vi "Write Trigger.vi"(8 "error in (no error)":errorcluster, 10 "PV":refnum<class "PV.lvclass">, 11 "PVConnection in":refnum<class "PVConnection.lvclass">) -> (0 "error out":errorcluster, 3 "PVConnection out":refnum<class "PVConnection.lvclass">)   [LabVIEW 2015, in "CS++ProcessVariables.lvlib" / "PVConnection.lvclass"]
doc: "Publish a process variable to trigger a paramater less message."
uses:
  PVConnection.lvclass
  ProcessVariable/PV.lvclass
  PVConnection.lvclass/PVConnection.ctl
  ProcessVariable/PV.lvclass/PV.ctl
  CS++BaseClasses/Base/CS++Base.lvclass/CS++Base.ctl
  Libraries/Utilities/CS++Utilities.lvlib
  CS++BaseClasses/Base/CS++Base.lvclass
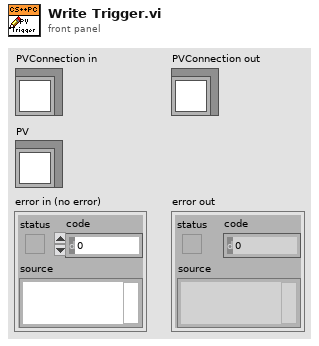
[diagram p1: front panel]
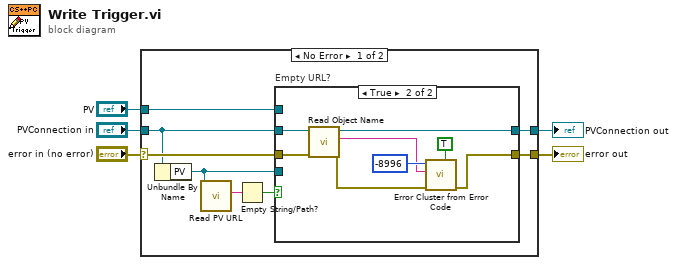
[diagram p0: block diagram]
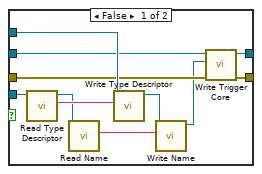
[diagram p2: hidden frame]
diagram:
  n1 = case shown="No Error" "error in (no error)" {
    selector: "error in (no error)" -> [w12 w34]
    tunnel: [w9 w34] -> w4
    tunnel: [w10 w33] -> w2
    tunnel: "PVConnection in" -> [w11 w33]
    tunnel: "PV" -> [w13 _]
    frame No Error {
      n2 = Unbundle By Name(w11) -> ("PV"=w7:refnum<class "PV.lvclass">)
      n3 = call "Read PV URL.vi"("PV in"=w7) -> ("PV URL"=w8:string)  [unwired: 8 in, 2 out]
      n4 = Empty String/Path?(string/path=w8) -> (empty?=w6:bool)
      n5 = case "Empty URL?" shown="True" w6 {
        tunnel: w13 -> [w24 _]
        tunnel: w12 -> [w19 w27]
        tunnel: w11 -> [w17 w29]
        tunnel: [w16 w28] -> w10
        tunnel: [w15 w30] -> w9
        tunnel: w7 -> [w14 _]
        frame False {
          n6 = call "Read Type Descriptor.vi"("PV in"=w14) -> ("Type Descriptor"=w23:string, "PV out"=w22:refnum<class "PV.lvclass">)  [unwired: 8 in, 1 out]
          n7 = call "Read Name.vi"("PV in"=w22) -> ("Name"=w21:string)  [unwired: 8 in, 2 out]
          n8 = call "Write Type Descriptor.vi"("Type Descriptor"=w23, "PV in"=w24) -> ("PV out"=w20:refnum<class "PV.lvclass">)  [unwired: 8 in, 1 out]
          n9 = call "Write Name.vi"("Name"=w21, "PV in"=w20) -> ("PV out"=w18:refnum<class "PV.lvclass">)  [unwired: 8 in, 1 out]
          n10 = call-dynamic "Write Trigger Core.vi"("error in (no error)"=w19, "PV"=w18, "PVConnection in"=w17) -> ("error out"=w15:errorcluster, "PVConnection out"=w16:refnum<class "PVConnection.lvclass">)  [unwired: 7 in]
        }
        frame True {
          n11 = call "Read Object Name.vi"("error in (no error)"=w27, "Base in"=w29) -> ("error out"=w26:errorcluster, "Object Name"=w25:string, "Base out"=w28:refnum<class "PVConnection.lvclass">)  [unwired: 7 in]
          n12 = call "Error Cluster from Error Code.vi"("is warning? (False)"=TRUE, "Error In"=w26, "Error Message (\"\")"=w25, "Error Code (0)"=-8996 ("error code (no error:0)")) -> ("Error Out"=w30:errorcluster)  [unwired: 7 in]
        }
      }
    }
    frame Error {
    }
  }
  "error out" <- w4
  "PVConnection out" <- w2
